vi "Shutdown.vi"(8 "Error In":errorcluster) -> (0 "Error Out":errorcluster)   [LabVIEW 2012]
uses:
  libs/LV-Utilities/LV-Utilities.lvlib
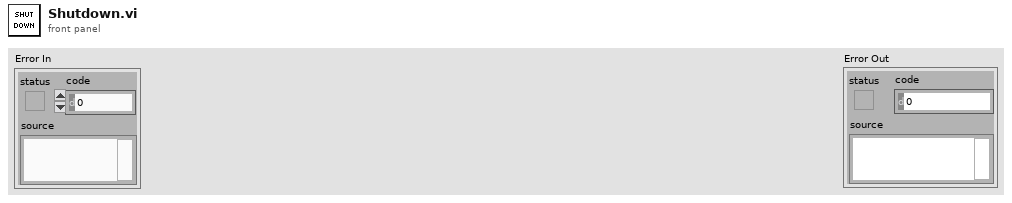
[diagram p1: front panel]
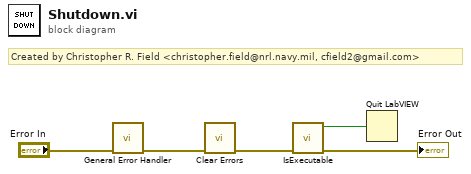
[diagram p0: block diagram]
diagram:
  # "Created by Christopher R. Field <christopher.field@nrl.navy.mil, cfield2@gmail.com>"
  n1 = call <vilib>:"General Error Handler.vi"("error in (no error)"="Error In") -> ("error out"=w3:errorcluster)  [unwired: 10 in, 4 out]
  n2 = call <vilib>:"Clear Errors.vi"("error in (no error)"=w3) -> ("error out"=w4:errorcluster)  [unwired: 6 in]
  n3 = call "IsExecutable.vi"("Error In"=w4) -> ("Error Out"=→"Error Out":errorcluster, "Executable?"=w5:bool)  [unwired: 9 in]
  n4 = Quit LabVIEW(quit? (T)=w5) -> ()
